vi "Function Gen Scan.vi"(8 "error in (no error)":errorcluster, 10 "Function Generator.lvclass":refnum<class "Function Generator.lvclass">, 11 "Function Gen Scan in":refnum<class "Function Gen Scan.lvclass">) -> (0 "error out":errorcluster, 3 "Function Gen Scan out":refnum<class "Function Gen Scan.lvclass">)   [LabVIEW 2023, in "Function Gen Scan.lvclass"]
uses:
  Function Gen Scan.lvclass
  C:/LabVIEW-programs/Scanners/Scanner/Scanner.lvclass
  Instruments/Function Generator/Function Generator.lvclass
  C:/LabVIEW-programs/Instruments/Utility Classes/Scannable/Scannable.lvclass
  Function Gen Scan.lvclass/Function Gen Scan.ctl
  Scanner/Scanner.lvclass
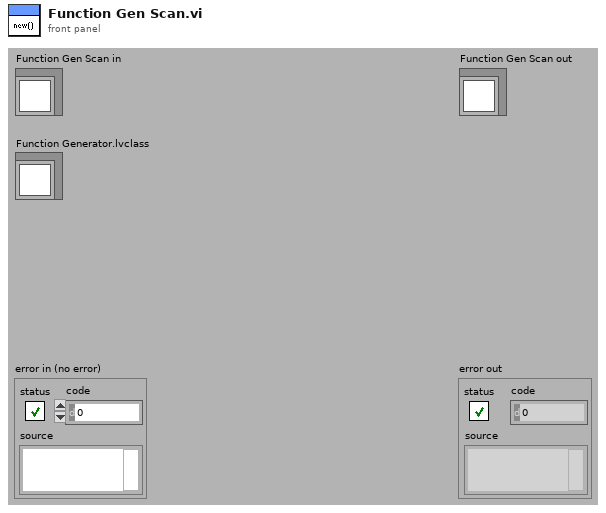
[diagram p1: front panel]
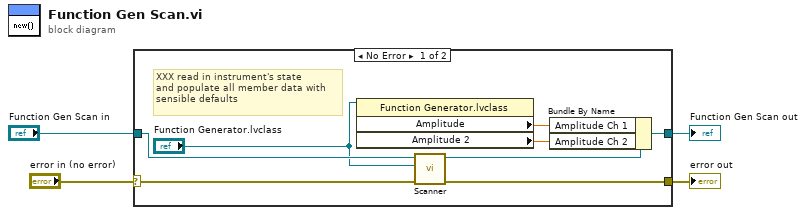
[diagram p0: block diagram]
diagram:
  n1 = case shown="No Error" "error in (no error)" {
    selector: "error in (no error)" -> [w10 w14]
    tunnel: [w9 w14] -> w3
    tunnel: [w7 w13] -> w1
    tunnel: "Function Gen Scan in" -> [w12 w13]
    frame No Error {
      # "XXX read in instrument's state\nand populate all member data with\nsensible defaults"
      n2 = property class="Function Generator.lvclass"(reference="Function Generator.lvclass") -> ("Amplitude"=w6:dbl[unit], "Amplitude 2"=w5:dbl[unit])  [unwired: 1 in, 2 out]
      n3 = call "Scanner.vi"("error in (no error)"=w10, "Scannable"="Function Generator.lvclass", "Scanner.lvclass in"=w12) -> ("error out"=w9:errorcluster, "Scanner.lvclass out"=w11:refnum<class "Function Gen Scan.lvclass">)  [unwired: 1 in, 6 out]
      n4 = Bundle By Name(cluster=w11, "Amplitude Ch 1"=w6, "Amplitude Ch 2"=w5) -> (w7:refnum<class "Function Gen Scan.lvclass">)
    }
    frame Error {
    }
  }
  "error out" <- w3
  "Function Gen Scan out" <- w1
